vi "ADCS.Get.ErrorByte.vi"(8 "error":errorcluster) -> (0 "error  out":errorcluster, 3 "Error Byte":u8)   [LabVIEW 2024, in "Diagnostics Addon Engine.lvlib"]
uses:
  Diagnostics Addon Engine.lvlib
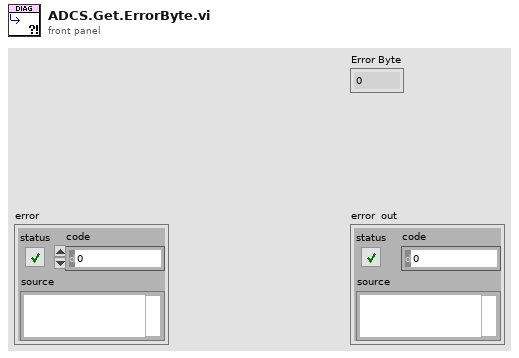
[diagram p1: front panel]
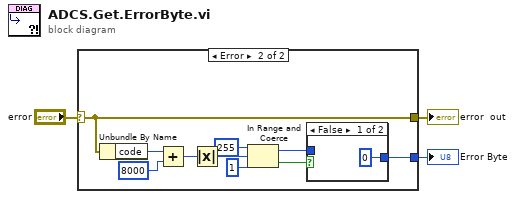
[diagram p0: block diagram]
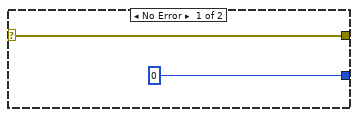
[diagram p2: hidden frame]
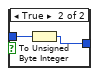
[diagram p3: hidden frame]
diagram:
  n1 = case shown="Error" "error" {
    selector: "error" -> [w4 w6]
    tunnel: [u8 0 w8] -> w3
    tunnel: [w4 w6] -> w2
    frame No Error {
    }
    frame Error {
      n2 = Unbundle By Name(w6) -> ("code"=w15:i32)
      n3 = Add(x=w15, y=8000) -> (x+y=w13:i32)
      n4 = Absolute Value(x=w13) -> (abs(x)=w12:i32)
      n5 = In Range and Coerce(upper limit=255, x=w12, lower limit=1) -> (coerced(x)=w7:i32, In Range?=w9:bool)
      n6 = case shown="False" w9 {
        tunnel: [u8 0 ("upper limit") w17] -> w8
        tunnel: w7 -> [_ w18]
        frame False {
        }
        frame True {
          n7 = To Unsigned Byte Integer(number=w18) -> (unsigned 8bit integer=w17:u8)
        }
      }
    }
  }
  "Error Byte" <- w3
  "error  out" <- w2
